vi "Apply DSF Configuration to Node.vi"(8 "error in (no error)":errorcluster, 10 "NewVal":path, 11 "Item Ref in":T1 format="%.0x") -> (0 "error out":errorcluster)   [LabVIEW 2017, in "Data Sharing Framework System Explorer.lvlib"]
uses:
  Data Sharing Framework System Explorer.lvlib
  <vilib>/NI Veristand/Custom Device API/Custom Device Item Ref.ctl
  <vilib>/NI Veristand/Custom Device API/Custom Device API.lvlib
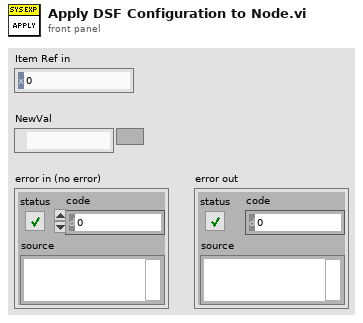
[diagram p1: front panel]
types:
  T1 = typedef "Custom Device API.lvlib/Custom Device Item Ref.ctl" = u64
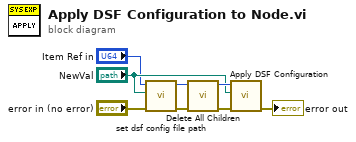
[diagram p0: block diagram]
diagram:
  n1 = call "set dsf config file path.vi"("error in (no error)"="error in (no error)", "Path"="NewVal", "Item Ref in"="Item Ref in") -> ("error out"=w6:errorcluster, "Item Ref out"=w5:T1)  [unwired: 7 in]
  n2 = call "Delete All Children.vi"("error in (no error)"=w6, "Item Ref in"=w5) -> ("error out"=w7:errorcluster, "Item Ref out"=w8:T1)  [unwired: 8 in]
  n3 = call "Apply DSF Configuration.vi"("error in (no error)"=w7, "path"="NewVal", "Item Ref in"=w8) -> ("error out"=→"error out":errorcluster)  [unwired: 8 in]
